vi "tcsshminitFlags.vi"(8 "error in (no error)":errorcluster) -> (0 "error out":errorcluster)   [LabVIEW 2016, in "SALLV_tcs.lvlib"]
doc: "void tcs_shm_initFlags();"
uses:
  SALLV_tcs.lvlib
  SALLV_tcs.so
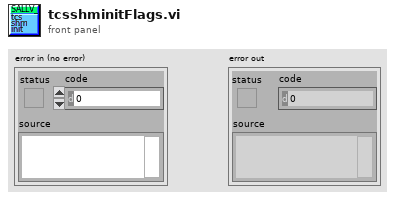
[diagram p1: front panel]
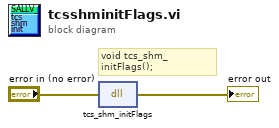
[diagram p0: block diagram]
diagram:
  # "void tcs_shm_initFlags();"
  n1 = dll-call lib="home/saluser/ct_tcs/ts_sallv_tcs/SALLV_tcs.*" fn="tcs_shm_initFlags"(error in="error in (no error)") -> (error out=→"error out":errorcluster)  [unwired: 3 in, 1 out]
